vi "microsec to sec.vi"(3 "data_timestamp us":i64) -> (1 "timestamp s":dbl format="%<%H:%M:%S%3u\n%m/%d/%Y>T")   [LabVIEW 2020, in "Vecto.lvlib"]
uses:
  Vecto.lvlib
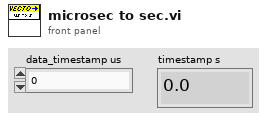
[diagram p1: front panel]
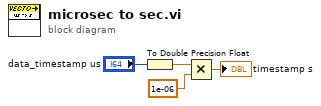
[diagram p0: block diagram]
diagram:
  n1 = To Double Precision Float(number="data_timestamp us") -> (double precision float=w3:dbl)
  n2 = Multiply(x=w3, y=1e-06) -> (x*y=→"timestamp s":dbl)
